vi "Parse CSV String (UTF-16).vi"(7 "delimiter (,) *ASCII":string=",", 10 "error in":errorcluster, 11 "CSV string *UTF-16":string) -> (2 "error out":errorcluster, 3 "2-D array *UTF-16":string[][](array[string]))   [LabVIEW 2013, in "SET_Robust CSV (UTF-16).lvlib"]
doc: "<b>http://en.wikipedia.org/wiki/Comma-separated_values</b>\n\nConvert a CSV (Character Separated Values) spreadsheet string to a 2D array of strings.\nThe input CSV spreadsheet string is assumed to be ANSI encoded and formatted in accordance with RFC-4180 (see <b>http://tools.ietf.org/html/rfc4180</b>). \nAll EOLs (CR, LF or CRLF) will be converted to LF and all escaped double quotes will be un-escaped in the output array.\n\nRev 0.3.0 02/20/2014 Ryan Porter\n- Added feature to replace all EOLs (0x0A, 0x0D) with LF (0x0A) so as to avoid adding a blank row when encountering CR+LF at the end of a line.\n- Added feature to allow any single character delimiter (not just the comma).\n- Removed the read text file and path terminals. \n- Changed Icon and connector pane layout.\n- Added error case structure around diagram.\n- Changed file name to Parse CSV String\n\nRev 0.2.0 06/08/2011 P. Brooks\n Added feature to replace opening and closing double quotes (0x93 & 0x94) with simple quote (0x22).\n\nRev 0.1.0 05/31/2011 P. Brooks\n Added option to handle strings. If CSV string is NULL (default) then the file in CSV File Path will be parsed instead of CSV string.\n\nRev 0.0.0 05/09/2011 P. Brooks\n Originated."
uses:
  SET_Robust CSV (UTF-16).lvlib
  Unicode/SET_Unicode Tools.lvlib
panel:
  # "Parse CSV String.vi\n\nConvert a CSV (Character Separated Values) spreadsheet string to a 2D array of strings.\nThe input CSV spreadsheet string is assumed to be ANSI encoded and formatted in accordance with RFC-4180 (see http://tools.ietf.org/html/rfc4180). \nAll EOLs (CR, LF or CRLF) will be converted to LF and all escaped double quotes will be un-escaped in the output array."
  # "Wikipedia Example Text \n(using opening and closing quotes)"
  # "Year,Make,Model,Description,Price\n1997,Ford,E350, “ac, abs, moon”,3000.00\n1999,Chevy,“Venture ““Extended Edition”””,“”,4900.00\n1999,Chevy,“ Venture ““ Extended Edition, Very Large”””,“”,5000.00\n1996,Jeep,Grand Cherokee,“MUST SELL!\nair, moon roof, loaded”,4799.00"
  # "http://en.wikipedia.org/wiki/Comma-separated_values"
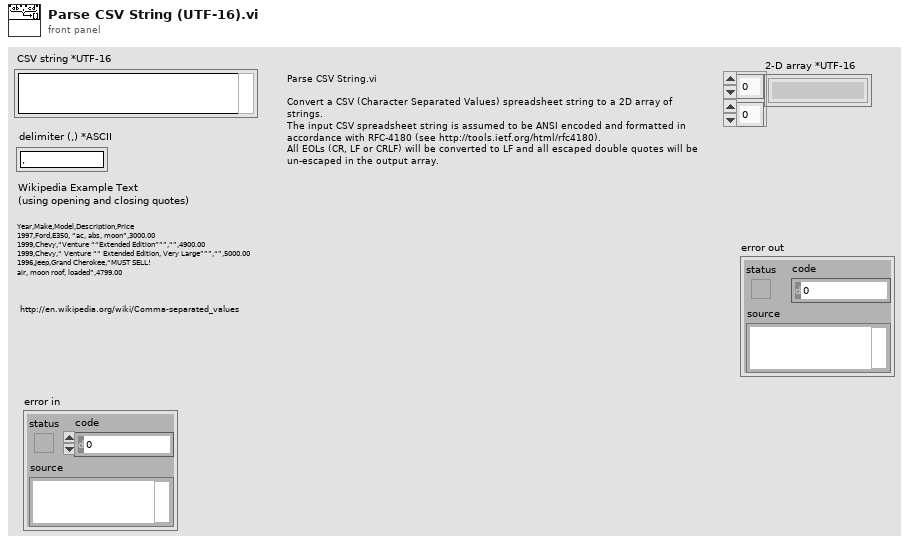
[diagram p1: front panel]
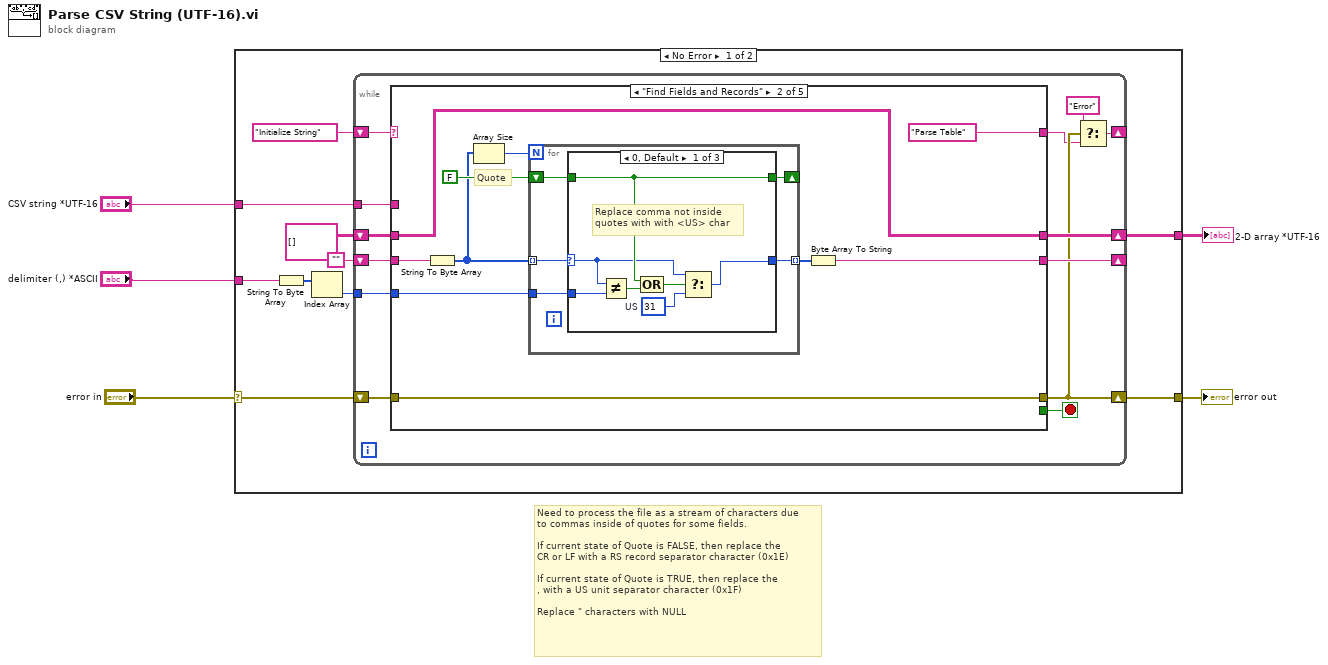
[diagram p0: block diagram]
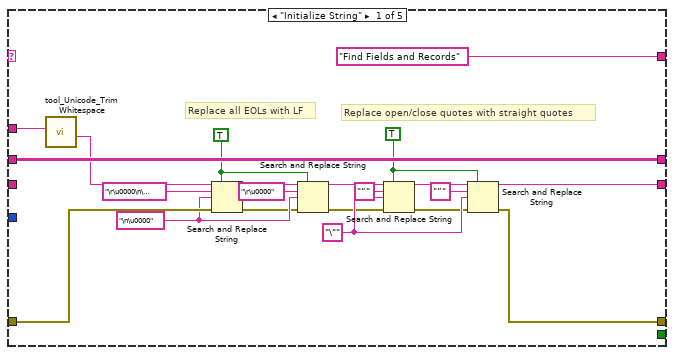
[diagram p2: hidden frame]
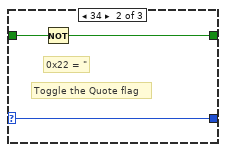
[diagram p3: hidden frame]
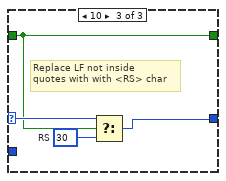
[diagram p4: hidden frame]
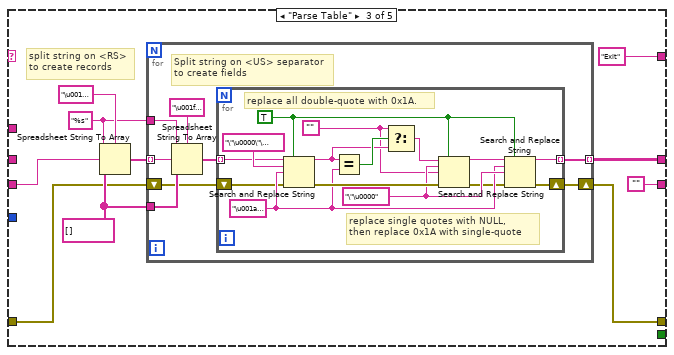
[diagram p5: hidden frame]
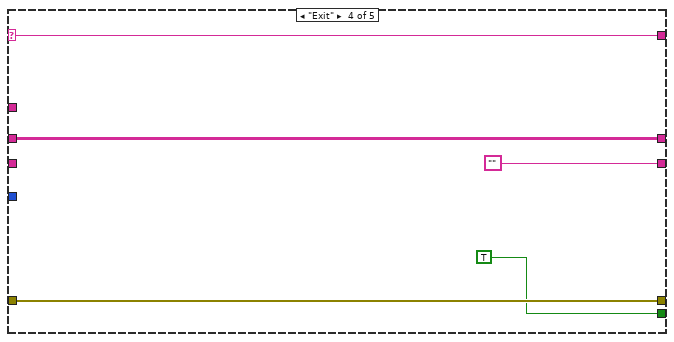
[diagram p6: hidden frame]
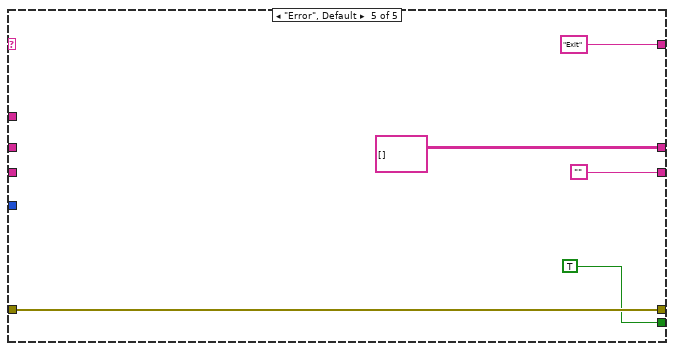
[diagram p7: hidden frame]
diagram:
  # "Need to process the file as a stream of characters due \nto commas inside of quotes for some fields.\n\nIf current state of Quote is FALSE, then replace the\nCR or LF with a RS record separator character (0x1E)\n\nIf current state of Quote is TRUE, then replace the\n, with a US unit separator character (0x1F)\n\nReplace \" characters with NULL"
  n1 = case shown="No Error" "error in" {
    selector: "error in" -> [w6 w122]
    tunnel: [w12 w122] -> w5
    tunnel: [w11 _] -> w4
    tunnel: "CSV string *UTF-16" -> [w10 _]
    tunnel: "delimiter (,) *ASCII" -> [w9 _]
    frame No Error {
      n2 = String To Byte Array(string=w9) -> (unsigned byte array=w8:u8[])
      n3 = Index Array(array=w8) -> (element=w7:u8)  [unwired: 1 in]
      n4 = while {
        shift-right: [w28] -> _
        shift-left: "" -> [w27]
        shift-right: [w19] -> _
        shift-left: "Initialize String" -> [w24]
        shift-right: [w26] -> w11
        shift-left: string[][] [] -> [w25]
        shift-right: [w22] -> w12
        shift-left: w6 -> [w23]
        tunnel: w10 -> [w17]
        tunnel: w7 -> [w16]
        stop <- w18 stop-if-true
        n5 = case shown="\"Find Fields and Records\"" w24 {
          selector: w24 -> [_ _ _ w115 _]
          tunnel: [w40 w54 "" "" ""] -> w28
          tunnel: ["Find Fields and Records" "Parse Table" "Exit" ("t") w115 "Exit" ("t")] -> w21
          tunnel: [_ _ _ TRUE TRUE] -> w18
          tunnel: w27 -> [_ w52 w80 _ _]
          tunnel: [w47 w53 w85 w112 string[][] []] -> w26
          tunnel: w25 -> [w47 w53 _ w112 _]
          tunnel: [w38 w50 w82 w116 w121] -> w22
          tunnel: w23 -> [w49 w50 w79 w116 w121]
          tunnel: w17 -> [w30 _ _ _ _]
          tunnel: w16 -> [_ w51 _ _ _]
          frame "Initialize String" {
            w34 = TRUE ("replace all? (F)")
            w33 = "\n\u0000" ("search string")
            w41 = TRUE ("replace all? (F)")
            w43 = "\"" ("replace string (\"\")")
            # "Replace open/close quotes with straight quotes"
            # "Replace all EOLs with LF"
            n6 = call "tool_Unicode_Trim Whitespace.vi"("String in *UTF-16"=w30) -> ("String out *UTF-16"=w29:string)  [unwired: 6 in]
            n7 = Search and Replace String(replace all?=w34, input string=w29, search string="\r\u0000\n\u0000", replace string=w33, error in=w49) -> (result string=w36:string, error out=w31:errorcluster)  [unwired: 3 in, 2 out]
            n8 = Search and Replace String(replace all?=w34, input string=w36, search string="\r\u0000", replace string=w33, error in=w31) -> (result string=w46:string, error out=w37:errorcluster)  [unwired: 3 in, 2 out]
            n9 = Search and Replace String(replace all?=w41, input string=w46, search string="“", replace string=w43, error in=w37) -> (result string=w44:string, error out=w39:errorcluster)  [unwired: 5 out]
            n10 = Search and Replace String(replace all?=w41, input string=w44, search string="”", replace string=w43, error in=w39) -> (result string=w40:string, error out=w38:errorcluster)  [unwired: 5 out]
          }
          frame "Find Fields and Records" {
            # "Quote"
            n11 = String To Byte Array(string=w52) -> (unsigned byte array=w57:u8[])
            n12 = Array Size(array=w57) -> (size(s)=w58:i32)
            n13 = for {
              N: w58 -> [_]
              tunnel: w57 -> [w62] mode=indexing
              shift-right: [w63] -> _
              shift-left: FALSE -> [w64]
              tunnel: [w61] -> w55 mode=indexing
              tunnel: w51 -> [w60]
              n14 = case shown="0, Default" w62 {
                selector: w62 -> [w65 w72 w76]
                tunnel: w64 -> [w68 w74 w75]
                tunnel: w60 -> [w70 _ _]
                tunnel: [w68 w73 w75] -> w63
                tunnel: [w71 w72 w77] -> w61
                frame 0, Default {
                  w66 = u8 31  # US
                  # "Replace comma not inside \nquotes with with <US> char"
                  n15 = Not Equal?(x=w65, y=w70) -> (x != y?=w69:bool)
                  n16 = Compound Arithmetic op=OR(w68, w69) -> (w67:bool)
                  n17 = Select(t=w65, s=w67, f=w66) -> (s? t:f=w71:u8)
                }
                frame 34 {
                  # "0x22 = \""
                  # "Toggle the Quote flag"
                  n18 = Not(x=w74) -> (.not. x?=w73:bool)
                }
                frame 10 {
                  w78 = u8 30  # RS
                  # "Replace LF not inside \nquotes with with <RS> char"
                  n19 = Select(t=w76, s=w75, f=w78) -> (s? t:f=w77:u8)
                }
              }
            }
            n20 = Byte Array To String(unsigned byte array=w55) -> (string=w54:string)
          }
          frame "Parse Table" {
            w88 = string[] []
            w83 = "%s" ("format string")
            # "split string on <RS>\nto create records"
            n21 = Spreadsheet String To Array(delimiter (Tab)="\u001e\u0000", format string=w83, spreadsheet string=w80, array type (2D Dbl)=w88) -> (array=w87:string[])
            n22 = for {
              tunnel: w87 -> [w96] mode=indexing
              tunnel: w88 -> [w93]
              tunnel: [w92] -> w85 mode=indexing
              tunnel: w83 -> [w91]
              shift-right: [w89] -> w82
              shift-left: w79 -> [w90]
              # "Split string on <US> separator\nto create fields"
              n23 = Spreadsheet String To Array(delimiter (Tab)="\u001f\u0000", format string=w91, spreadsheet string=w96, array type (2D Dbl)=w93) -> (array=w94:string[])
              n24 = for {
                tunnel: w94 -> [w98] mode=indexing
                tunnel: [w99] -> w92 mode=indexing
                shift-right: [w100] -> w89
                shift-left: w90 -> [w102]
                w97 = ""
                w107 = "\"\u0000" ("input string")
                w108 = TRUE ("replace all? (F)")
                w106 = "\u001a\u0000" ("replace string (\"\")")
                # "replace single quotes with NULL,\nthen replace 0x1A with single-quote"
                # "replace all double-quote with 0x1A."
                n25 = Search and Replace String(replace all?=w108, input string=w98, search string="\"\u0000\"\u0000", replace string=w106, error in=w102) -> (result string=w104:string, error out=w110:errorcluster)  [unwired: 5 out]
                n26 = Equal?(x=w104, y=w106) -> (x = y?=w105:bool)
                n27 = Select(t=w97, s=w105, f=w104) -> (s? t:f=w103:string)
                n28 = Search and Replace String(replace all?=w108, input string=w103, search string=w107, replace string=w97, error in=w110) -> (result string=w109:string, error out=w101:errorcluster)  [unwired: 5 out]
                n29 = Search and Replace String(replace all?=w108, input string=w109, search string=w106, replace string=w107, error in=w101) -> (result string=w99:string, error out=w100:errorcluster)  [unwired: 1 in, 4 out]
              }
            }
          }
          frame "Exit" {
          }
          frame "Error", Default {
          }
        }
        n30 = Select(t="Error", s=w22, f=w21) -> (s? t:f=w19:string)
      }
    }
    frame Error {
    }
  }
  "error out" <- w5
  "2-D array *UTF-16" <- w4
